vi "New_S2C_FORNAX_Proc_ManageVipFile.vi"(8 "Error In":errorcluster, 11 "Data In":string) -> (0 "Error Out":errorcluster, 3 "Data Out":string[](array[string]))   [LabVIEW 2015]
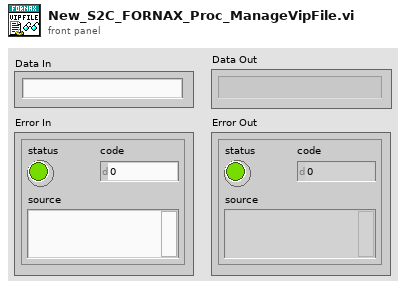
[diagram p1: front panel]
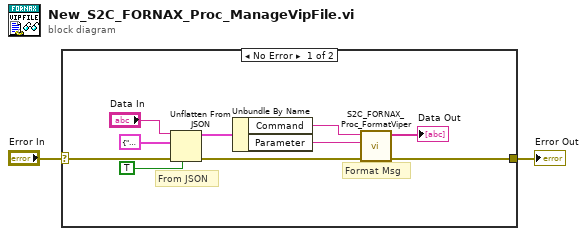
[diagram p0: block diagram]
diagram:
  n1 = case shown="No Error" "Error In" {
    selector: "Error In" -> [w11 w13]
    tunnel: [w9 w13] -> w1
    frame No Error {
      # "Format Msg"
      # "From JSON"
      n2 = Unflatten From JSON(JSON string="Data In", type and defaults=cluster{"Command":string, "Parameter":string} {"Command"="", "Parameter"=""}, default null elements? (F)=TRUE, error in (no error)=w11) -> (value=w8:cluster{"Command":string, "Parameter":string}, error out=w4:errorcluster)  [unwired: 3 in]
      n3 = Unbundle By Name(w8) -> ("Command"=w3:string, "Parameter"=w5:string)
      n4 = call "S2C_FORNAX_Proc_FormatViper.vi"("Error In"=w4, "Parameter"=w5, "Command"=w3) -> ("Error Out"=w9:errorcluster, "VipMsg"=→"Data Out":string[])  [unwired: 7 in]
    }
    frame Error {
    }
  }
  "Error Out" <- w1
